vi "CLI.git.vi"(8 "error in (no error)":errorcluster, 9 "Option":string="start", 10 "Command":T1="config", 11 "Git in":refnum<class "Git.lvclass">) -> (0 "error out":errorcluster, 1 "standard error":string, 2 "standard output":string, 3 "Git out":refnum<class "Git.lvclass">, 4 "return code":i32)   [LabVIEW 2019, in "Git.lvclass"]
uses:
  Git.lvclass
  Typedefs/Commands.git--combo.ctl
  Git.lvclass/Git.ctl
panel:
  # "Fatal: Not a git repository"
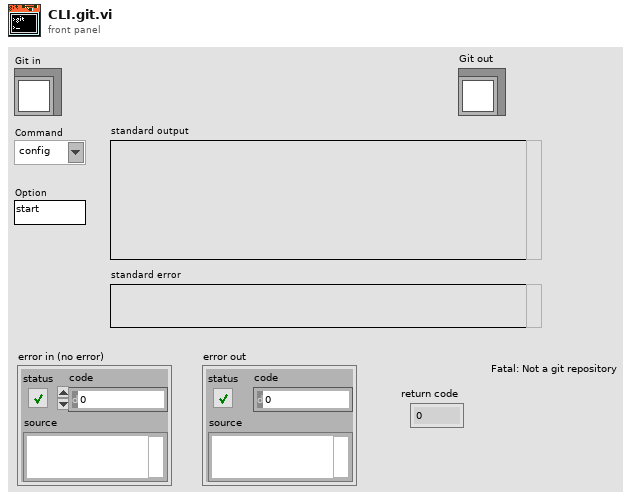
[diagram p1: front panel]
types:
  T1 = typedef "Git.lvclass/Commands.git--combo.ctl" = string
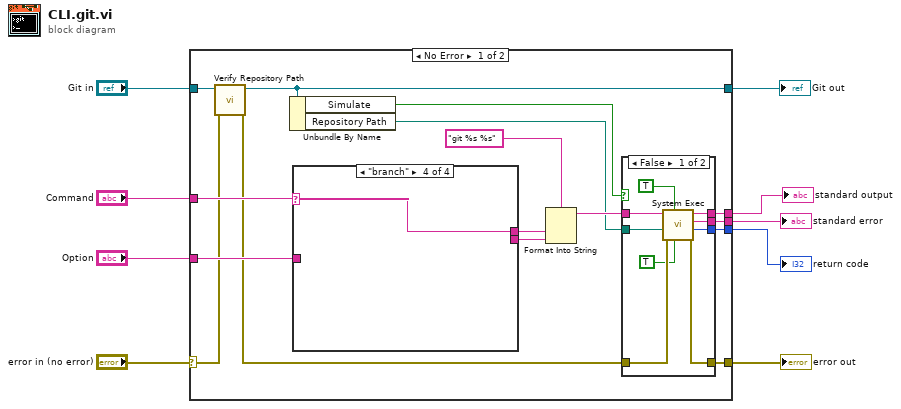
[diagram p0: block diagram]
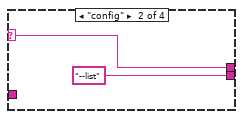
[diagram p4: hidden frame]
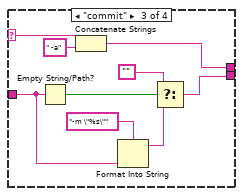
[diagram p5: hidden frame]
diagram:
  n1 = case shown="No Error" "error in (no error)" {
    selector: "error in (no error)" -> [w13 w51]
    tunnel: [w25 _] -> w9
    tunnel: [w24 w51] -> w8
    tunnel: "Option" -> [w23 _]
    tunnel: "Command" -> [w22 _]
    tunnel: [w21 _] -> w5
    tunnel: [w20 _] -> w4
    tunnel: "Git in" -> [w19 w50]
    tunnel: [w17 w50] -> w2
    frame No Error {
      n2 = call "Verify Repository Path.vi"("error in (no error)"=w13, "Git in"=w19) -> ("error out"=w18:errorcluster, "Git out"=w17:refnum<class "Git.lvclass">)  [unwired: 8 in]
      n3 = Unbundle By Name(w17) -> ("Simulate"=w10:bool, "Repository Path"=w14:path)
      n4 = case shown="\"branch\"" w22 {
        selector: w22 -> [w37 w39 w47 w49]
        tunnel: w23 -> [_ _ w44 _]
        tunnel: [w37 w39 w40 w49] -> w12
        tunnel: [_ "--list" w41 _] -> w11
        frame "status", Default {
        }
        frame "config" {
        }
        frame "commit" {
          n5 = Empty String/Path?(string/path=w44) -> (empty?=w46:bool)
          n6 = Concatenate Strings(w47, " -a" ("string")) -> (w40:string)
          n7 = Format Into String(format string="-m \"%s\"", w44) -> (resulting string=w43:string)  [unwired: 2 in, 1 out]
          n8 = Select(t="", s=w46, f=w43) -> (s? t:f=w41:string)
        }
        frame "branch" {
        }
      }
      n9 = Format Into String(format string="git %s %s", w12, w11) -> (resulting string=w16:string)  [unwired: 2 in, 1 out]
      n10 = case shown="False" w10 {
        tunnel: [w34 w36] -> w25
        tunnel: [w26 w35] -> w24
        tunnel: [w33 _] -> w21
        tunnel: [w32 _] -> w20
        tunnel: w18 -> [w31 w35]
        tunnel: w16 -> [w28 w36]
        tunnel: w14 -> [w27 _]
        frame False {
          n11 = call <vilib>:"System Exec.vi"("run minimized? (F)"=TRUE, "wait until completion? (T)"=TRUE, "error in (no error)"=w31, "working directory"=w27, "command line"=w28) -> ("error out"=w26:errorcluster, "return code"=w32:i32, "standard error"=w33:string, "standard output"=w34:string)  [unwired: 3 in]
        }
        frame True {
        }
      }
    }
    frame Error {
    }
  }
  "standard output" <- w9
  "standard error" <- w5
  "return code" <- w4
  "error out" <- w8
  "Git out" <- w2
